vi "Write directory.vi"(8 "error in (no error)":errorcluster, 10 "log dir":path, 11 "Log File in":refnum<class "Log File.lvclass">) -> (0 "error out":errorcluster, 3 "Log File out":refnum<class "Log File.lvclass">)   [LabVIEW 2018, in "Log File.lvclass"]
uses:
  Log File.lvclass
  Log File.lvclass/Log File.ctl
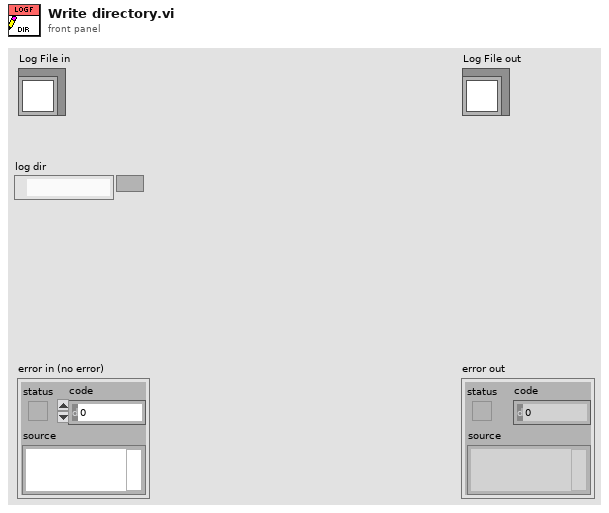
[diagram p1: front panel]
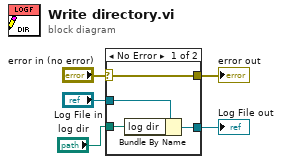
[diagram p0: block diagram]
diagram:
  n1 = case shown="No Error" "error in (no error)" {
    selector: "error in (no error)" -> [w7 w10]
    tunnel: [w7 w10] -> w4
    tunnel: [w8 w11] -> w2
    tunnel: "Log File in" -> [w9 w11]
    tunnel: "log dir" -> [w6 _]
    frame No Error {
      n2 = Bundle By Name(cluster=w9, "log dir"=w6) -> (w8:refnum<class "Log File.lvclass">)
    }
    frame Error {
    }
  }
  "error out" <- w4
  "Log File out" <- w2
